vi "QCA - DUT Transmit.vi"(0 "CART TCP Connection In":refnum<k5>, 5 "TV Parameters(DataType)":T1 {"Tx_Chan" format="%.0x"; "Standard" items=["80211A/G/J/P OFDM", "80211B/G DSSS", "80211G DSSSOFDM", "80211N MIMOOFDM", "80211AC MIMOOFDM"]; "OFDM Data Rate (Mbps)" items=["6", "9", "12", "18", "24", "36", "48", "54"]; "80211n PLCP Frame Format" items=["Mixed Format", "Greenfield Format"]; "FEC Coding Type" items=["BCC", "LDPC"]; "DSSS Data Rate (Mbps)" items=["1", "2", "5.5 CCK", "5.5 PBCC", "11 CCK", "11 PBCC", "22", "33"]}, 11 "error in (no error)":errorcluster) -> (4 "CART TCP Connection Out":refnum<k5>, 6 "Messages Logged":string[](array[string]), 14 "Command Sent":string, 15 "error out":errorcluster)   [LabVIEW 2011]
uses:
  TV/RW/Includes/WLAN - TV - RW - INC - TV_DataType_Cluster.ctl
  Controls/Transmit Config.ctl
  Controls/Data Rates.ctl
  Controls/Inter Frame Spacing modes.ctl
  Controls/Parameter.ctl
panel:
  out "32bit integer":i32
  in  "OFDM Data Rate (Mbps)":i32(ring) items=["6", "9", "12", "18", "24", "36", "48", "54"]
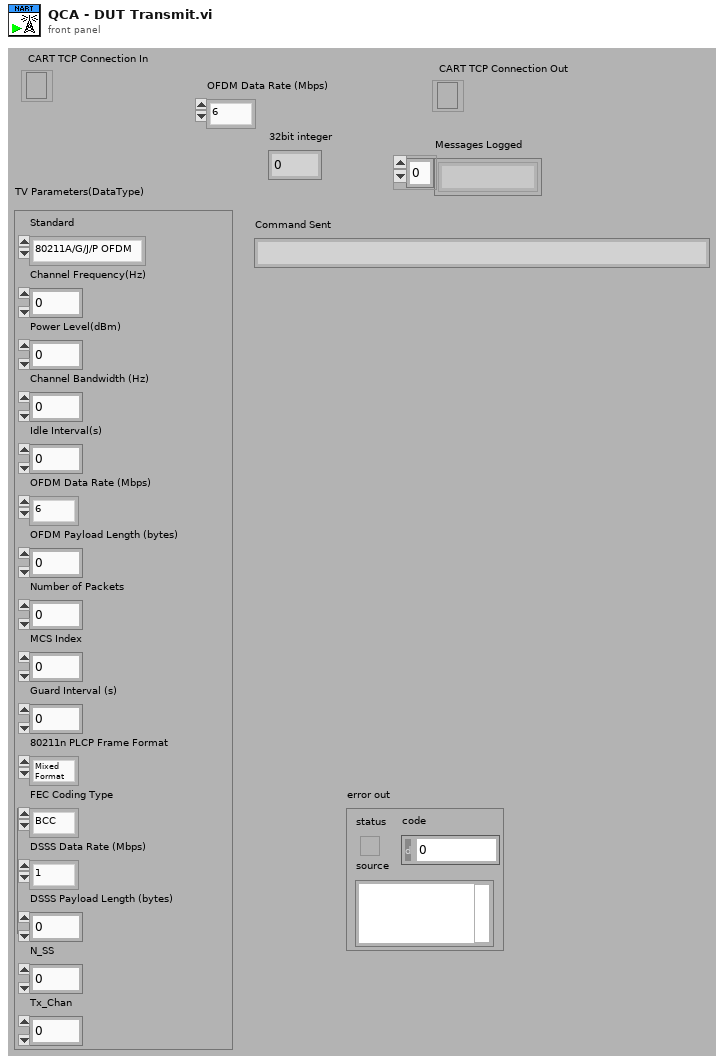
[diagram p1: front panel]
types:
  T1 = typedef "WLAN - TV - RW - INC - TV_DataType_Cluster.ctl" = cluster{"Standard":i32, "Channel Frequency(Hz)":dbl, "Power Level(dBm)":dbl, "Channel Bandwidth (Hz)":dbl, "Idle Interval(s)":dbl, "OFDM Data Rate (Mbps)":i32, "OFDM Payload Length (bytes)":i32, "Number of Packets":i32, "MCS Index":i32, "Guard Interval (s)":dbl, "80211n PLCP Frame Format":i32, "FEC Coding Type":i32, "DSSS Data Rate (Mbps)":i32, "DSSS Payload Length (bytes)":i32, "N_SS":i32, "Tx_Chan":u32}
  T2 = typedef "Data Rates.ctl" = string
  T3 = typedef "Transmit Config.ctl" = cluster{"Packet Length":u32, "Packet Count":i32, "Data Rate":T2, "Frequency, MHz":u32, "Continuous Frames":bool, "TX Power, dB":dbl}
  T4 = enum16{"none", "combined", "isolated", "iterate-combined ", "iterate-isolated"}
  T5 = typedef "Parameter.ctl" = cluster{"Name":string, "Type":enum16{"decimal", "string", "float", "hex"}}
  T6 = typedef "Inter Frame Spacing modes.ctl" = i16
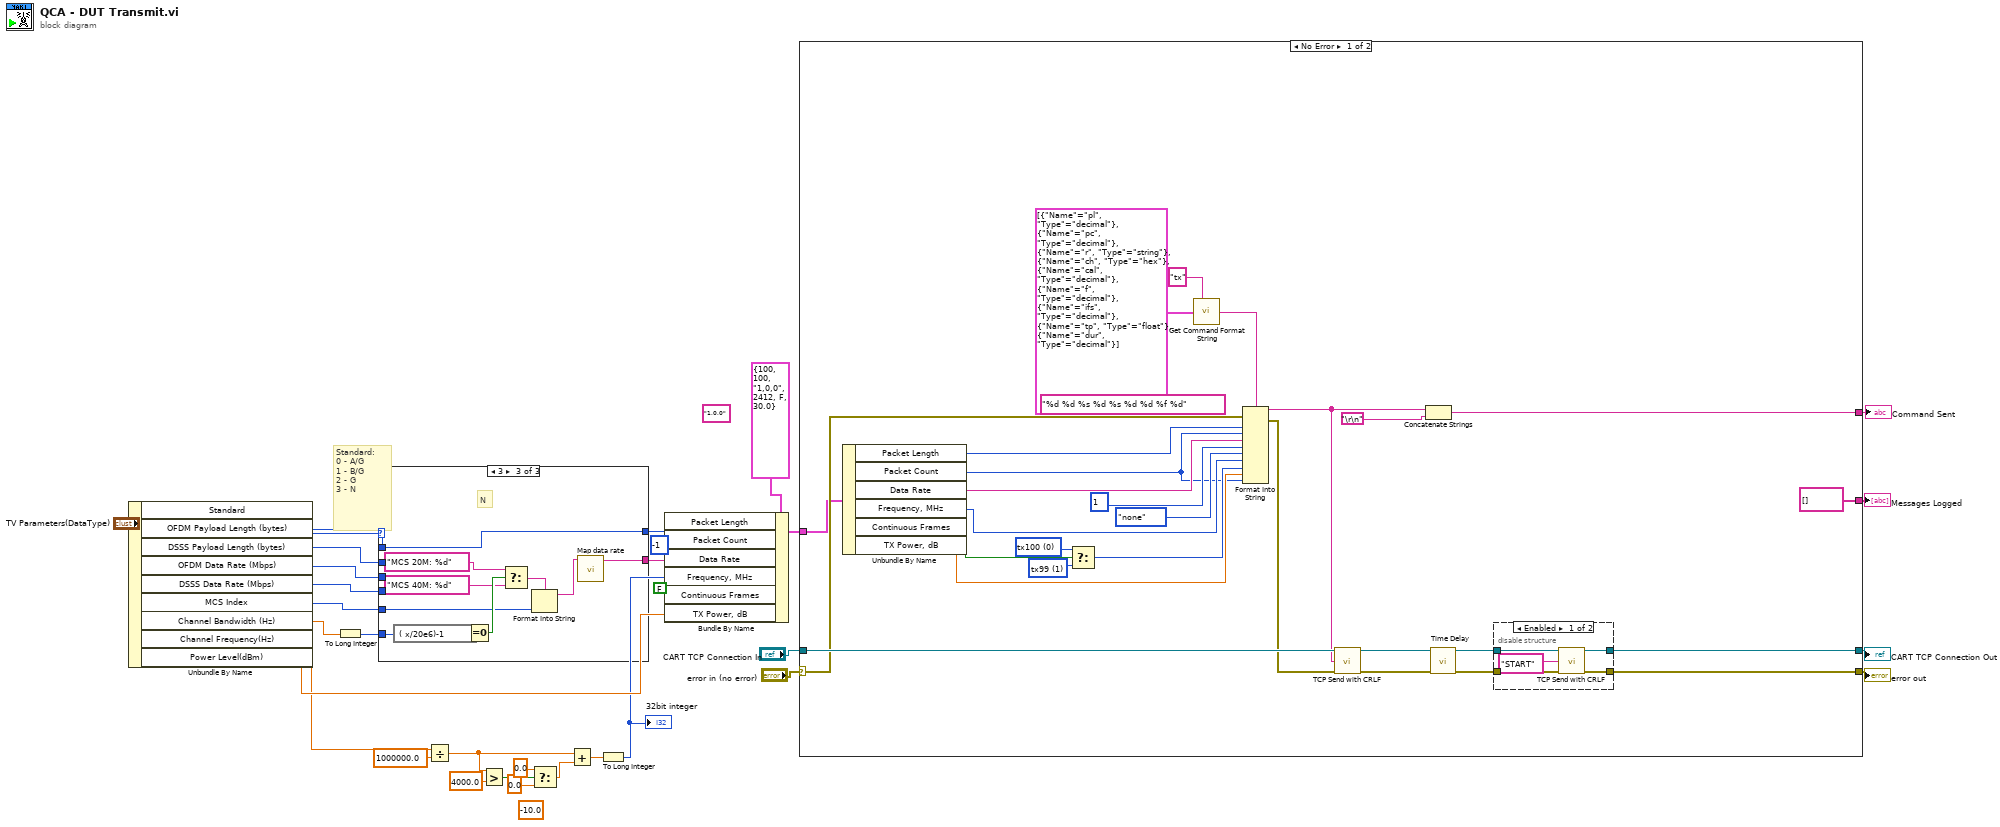
[diagram p0: block diagram]
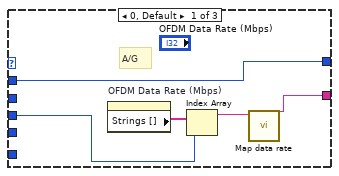
[diagram p2: hidden frame]
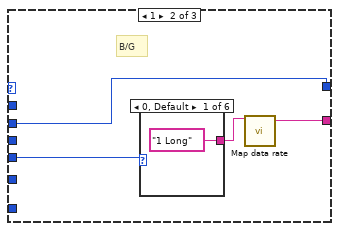
[diagram p3: hidden frame]
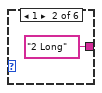
[diagram p4: hidden frame]
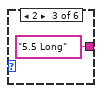
[diagram p5: hidden frame]
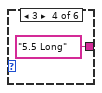
[diagram p6: hidden frame]
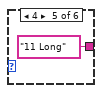
[diagram p7: hidden frame]
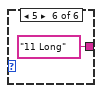
[diagram p8: hidden frame]
diagram:
  (unwired) -10.0 ("t")
  (unwired) T2 "1,0,0" ("Data Rate")
  # "Standard:\n0 - A/G\n1 - B/G\n2 - G\n3 - N"
  n1 = Unbundle By Name("TV Parameters(DataType)") -> ("Standard"=w21:i32, "OFDM Payload Length (bytes)"=w19:i32, "DSSS Payload Length (bytes)"=w18:i32, "OFDM Data Rate (Mbps)"=w17:i32, "DSSS Data Rate (Mbps)"=w15:i32, "MCS Index"=w14:i32, "Channel Bandwidth (Hz)"=w10:dbl, "Channel Frequency(Hz)"=w12:dbl, "Power Level(dBm)"=w16:dbl)
  n2 = To Long Integer(number=w10) -> (32bit integer=w9:i32)
  n3 = case shown="3" w21 {
    tunnel: [w37 w41 w57] -> w20
    tunnel: w19 -> [w37 _ w57]
    tunnel: w18 -> [_ w41 _]
    tunnel: w17 -> [w33 _ _]
    tunnel: w15 -> [_ w40 _]
    tunnel: w14 -> [_ _ w48]
    tunnel: [w36 w39 w56] -> w13
    tunnel: w9 -> [_ _ w49]
    frame 0, Default {
      # "A/G"
      n4 = property on="OFDM Data Rate (Mbps)" class="Ring (strict)"() -> ("Strings []"=w35:string[])  [unwired: 2 in, 2 out]
      n5 = Index Array(array=w35, index=w33) -> (element=w34:string)
      n6 = call "Map data rate.vi"("Data Rate In"=w34) -> ("Data Rate Out"=w36:string)  [unwired: 10 in]
    }
    frame 1 {
      # "B/G"
      n7 = case shown="0, Default" w40 {
        tunnel: ["1 Long" ("Data Rate In") "2 Long" ("Data Rate In") "5.5 Long" ("Data Rate In") "5.5 Long" ("Data Rate In") "11 Long" ("Data Rate In") "11 Long" ("Data Rate In")] -> w38
        frame 0, Default {
        }
        frame 1 {
        }
        frame 2 {
        }
        frame 3 {
        }
        frame 4 {
        }
        frame 5 {
        }
      }
      n8 = call "Map data rate.vi"("Data Rate In"=w38) -> ("Data Rate Out"=w39:string)  [unwired: 10 in]
    }
    frame 3 {
      # "N"
      n9 = expression code="( x/20e6)-1"(w49) -> (w53:i32)
      n10 = Equal To 0?(x=w53) -> (x = 0?=w54:bool)
      n11 = Select(t="MCS 20M: %d" ("format string"), s=w54, f="MCS 40M: %d" ("format string")) -> (s? t:f=w55:string)
      n12 = Format Into String(format string=w55, w48) -> (resulting string=w50:string)  [unwired: 2 in, 1 out]
      n13 = call "Map data rate.vi"("Data Rate In"=w50) -> ("Data Rate Out"=w56:string)  [unwired: 10 in]
    }
  }
  n14 = Divide(x=w12, y=1000000.0 ("x")) -> (x/y=w2:dbl)
  n15 = Greater?(x=w2, y=4000.0) -> (0:w8:bool)
  n16 = Select(t=0.0, s=w8, f=0.0) -> (s? t:f=w5:dbl)
  n17 = Add(x=w2, y=w5) -> (x+y=w1:dbl)
  n18 = To Long Integer(number=w1) -> (32bit integer=w4:i32)
  "32bit integer" <- w4
  n19 = Bundle By Name(cluster=T3 {"Packet Length"=100, "Packet Count"=100, "Data Rate"="1,0,0", "Frequency, MHz"=2412, "Continuous Frames"=FALSE, "TX Power, dB"=30.0} ("Transmit Config"), "Packet Length"=w20, "Packet Count"=-1, "Data Rate"=w13, "Frequency, MHz"=w4, "Continuous Frames"=FALSE, "TX Power, dB"=w16) -> (w25:T3)
  n20 = case shown="No Error" "error in (no error)" {
    selector: "error in (no error)" -> [w83 w93]
    tunnel: [w79 w93] -> w31
    tunnel: "CART TCP Connection In" -> [w84 w92]
    tunnel: [w80 w92] -> w29
    tunnel: [string[] [] ("Messages Logged") _] -> w28
    tunnel: [w71 _] -> w27
    tunnel: w25 -> [w58 _]
    frame No Error {
      (unwired) "%d %d %s %d %s %d %d %f %d" ("format string")
      w65 = T6 1 items=["Regular"=-1, "tx100"=0, "tx99"=1] ("ART2 Data.Transmit Config.Inter Frame Spacing")
      w66 = T6 0 items=["Regular"=-1, "tx100"=0, "tx99"=1] ("ART2 Data.Transmit Config.Inter Frame Spacing")
      n21 = Unbundle By Name(w58) -> ("Packet Length"=w81:u32, "Packet Count"=w62:i32, "Data Rate"=w69:T2, "Frequency, MHz"=w74:u32, "Continuous Frames"=w64:bool, "TX Power, dB"=w72:dbl)
      n22 = Select(t=w66, s=w64, f=w65) -> (s? t:f=w63:T6)
      n23 = call "Get Command Format String.vi"("Command"="tx", "Parameters"=T5[] [{"Name"="pl", "Type"=enum."decimal"}, {"Name"="pc", "Type"=enum."decimal"}, {"Name"="r", "Type"=enum."string"}, {"Name"="ch", "Type"=enum."hex"}, {"Name"="cal", "Type"=enum."decimal"}, {"Name"="f", "Type"=enum."decimal"}, {"Name"="ifs", "Type"=enum."decimal"}, {"Name"="tp", "Type"=enum."float"}, {"Name"="dur", "Type"=enum."decimal"}]) -> ("Command Format String"=w73:string)  [unwired: 13 in]
      n24 = Format Into String(format string=w73, error in=w83, w81, w62, w69, u32 1 ("Chains"), T4."none" ("input 5"), w74, w63, w72, w62) -> (resulting string=w61:string, error out=w82:errorcluster)  [unwired: 1 in]
      n25 = call "TCP Send with CRLF.vi"("CART TCP Connection"=w84, "data in"=w61, "error IO"=w82) -> ("CART TCP Connection Out"=w78:refnum<k5>, "error out"=w77:errorcluster)  [unwired: 11 in]
      n26 = Concatenate Strings(w61, "\r\n") -> (w71:string)
      n27 = call "Time Delay"("error in (no error)"=w77) -> ("error out"=w60:errorcluster)  [unwired: 10 in]
      n28 = disable-structure shown="Enabled" {
        disable-tunnel: w78 -> [w89 w91]
        disable-tunnel: [w88 w90] -> w79
        disable-tunnel: [w87 w91] -> w80
        disable-tunnel: w60 -> [w86 w90]
        frame Enabled {
          n29 = call "TCP Send with CRLF.vi"("CART TCP Connection"=w89, "data in"="START" ("format string"), "error IO"=w86) -> ("CART TCP Connection Out"=w87:refnum<k5>, "error out"=w88:errorcluster)  [unwired: 11 in]
        }
        frame Disabled {
        }
      }
    }
    frame Error {
    }
  }
  "error out" <- w31
  "CART TCP Connection Out" <- w29
  "Messages Logged" <- w28
  "Command Sent" <- w27
